vi "CloseCommunications .vi"(8 "error in (no error)":errorcluster, 11 "StepMotor in":refnum<class "StepMotor.lvclass">) -> (0 "error out":errorcluster, 3 "StepMotor out":refnum<class "StepMotor.lvclass">)   [LabVIEW 2010, in "StepMotor.lvclass"]
doc: "Закрытие соединения (связи) привода СПШ"
uses:
  StepMotor.lvclass
  StepMotor.lvclass/StepMotor.ctl
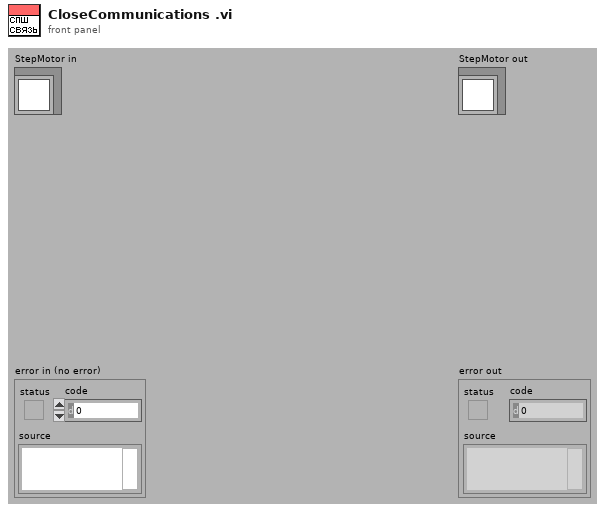
[diagram p1: front panel]
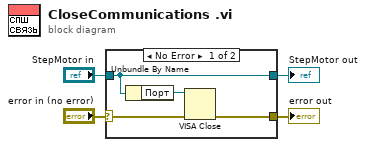
[diagram p0: block diagram]
diagram:
  n1 = case shown="No Error" "error in (no error)" {
    selector: "error in (no error)" -> [w7 w10]
    tunnel: [w5 w10] -> w3
    tunnel: [w8 w9] -> w1
    tunnel: "StepMotor in" -> [w8 w9]
    frame No Error {
      n2 = Unbundle By Name(w8) -> ("Порт"=w6:refnum<visa-resource-name>)
      n3 = VISA Close(VISA resource name=w6, error in (no error)=w7) -> (error out=w5:errorcluster)
    }
    frame Error {
    }
  }
  "error out" <- w3
  "StepMotor out" <- w1
